vi "Clear Log.vi"(8 "error in (no error)":errorcluster, 10 "Actor Q":refnum<class "Message Enqueuer.lvclass">, 11 "Message Logger in":refnum<class "Classic Logger.lvclass">) -> (0 "error out":errorcluster, 3 "Message Logger out":refnum<class "Classic Logger.lvclass">)   [LabVIEW 2017, in "MGI-Monitored Actor.lvlib" / "Classic Logger.lvclass"]
doc: "Clears the log for the specified actor\n\nCopyright: MGI 2016\nAuthor: Derek Trepanier"
uses:
  Classic Logger.lvclass
  <vilib>/ActorFramework/Message Enqueuer/Message Enqueuer.lvclass
  Monitor Data.ctl
  Classic Logger.lvclass/Classic Logger.ctl
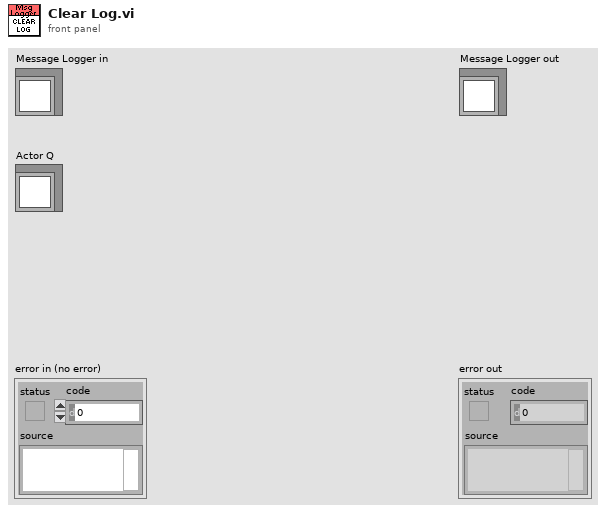
[diagram p1: front panel]
types:
  T1 = typedef "MGI-Monitored Actor.lvlib/Classic Logger.lvclass/Monitor Data.ctl" = cluster{"Time Stamp":timestamp, "class name":string, "Msg XML":string}
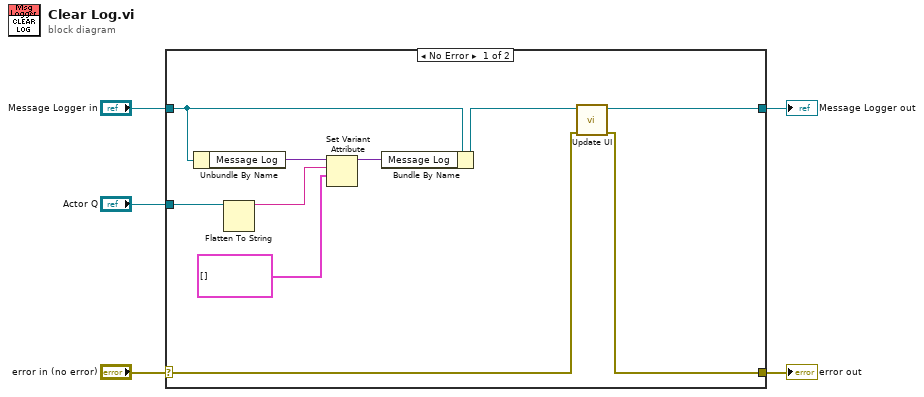
[diagram p0: block diagram]
diagram:
  n1 = case shown="No Error" "error in (no error)" {
    selector: "error in (no error)" -> [w7 w17]
    tunnel: [w8 w17] -> w4
    tunnel: [w9 w16] -> w2
    tunnel: "Message Logger in" -> [w15 w16]
    tunnel: "Actor Q" -> [w14 _]
    frame No Error {
      n2 = Unbundle By Name(w15) -> ("Message Log"=w13:variant)
      n3 = Flatten To String(anything=w14) -> (data string=w10:string)  [unwired: 3 in, 2 out]
      n4 = Set Variant Attribute(Variant=w13, name=w10, value=T1[] []) -> (Variant out=w11:variant)  [unwired: 1 in, 2 out]
      n5 = Bundle By Name(cluster=w15, "Message Log"=w11) -> (w12:refnum<class "Classic Logger.lvclass">)
      n6 = call "Update UI.vi"("error in (no error)"=w7, "Message Logger in"=w12) -> ("error out"=w8:errorcluster, "Message Logger out"=w9:refnum<class "Classic Logger.lvclass">)  [unwired: 8 in]
    }
    frame Error {
    }
  }
  "error out" <- w4
  "Message Logger out" <- w2
